vi "G_read.vi"() -> ()   [LabVIEW 2012]
panel:
  out "NAV":dbl[](array[numeric])
  out "Laser 2":u16[](array[numeric])
  out "Laser 1":u16[](array[numeric])
  out "RIONAV":dbl[](array[numeric])
  out "GPS 2 bestvel":u8[](array[numeric])
  out "GPS 1 bestvel":u8[](array[numeric])
  out "GPS 2 bestpos":u8[](array[numeric])
  out "GPS 1 bestpos":u8[](array[numeric])
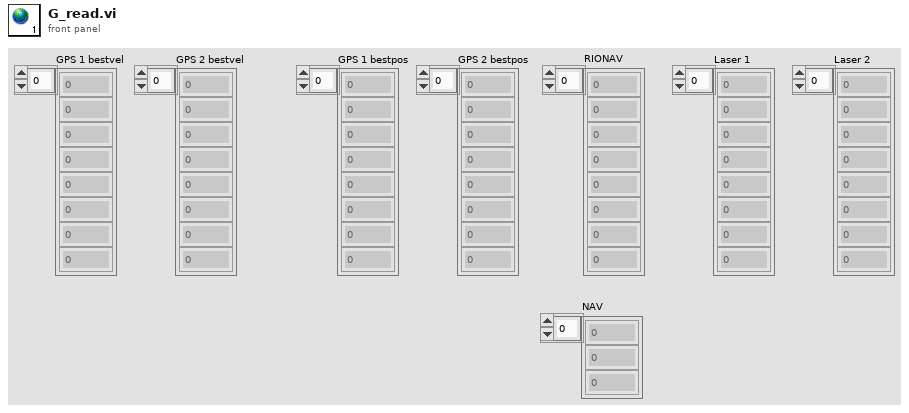
[diagram p1: front panel]
diagram:
